vi "限幅器（VAR）.vi"(3 "下限":variant, 4 "X_in":variant, 5 "上限":variant) -> (1 "X_Out":variant)   [LabVIEW 2012]
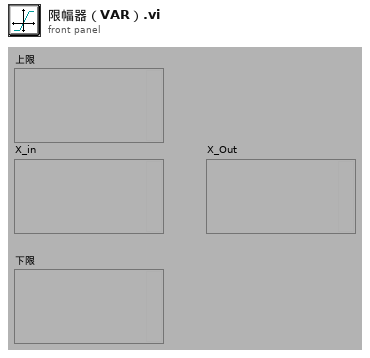
[diagram p1: front panel]
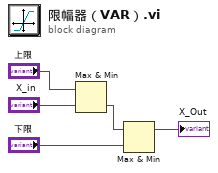
[diagram p0: block diagram]
diagram:
  n1 = Max & Min(x="上限", y="X_in") -> (min(x,y)=w3:variant)  [unwired: 1 out]
  n2 = Max & Min(x=w3, y="下限") -> (max(x,y)=→"X_Out":variant)  [unwired: 1 out]
